vi "SR430_init.vi"(0 "GPIB address":T1, 1 "triggeLevel [V]":dbl format="%.2f", 2 "triggerSlope":bool, 3 "discriminatorLevel [V]":dbl format="%.2f", 4 "discriminatorSlope":bool, 5 "error in (no error)":errorcluster, 7 "cursorOn":bool, 9 "useExternalClock":bool) -> (14 "GPIB address out":T1, 19 "error out":errorcluster)   [LabVIEW 2015, in "SR430Driver.lvlib"]
doc: "Initializes the SR430 \n\nCopyright (C)\nGesellschaft für Schwerionenforschung, GSI\nPlanckstr. 1\n64291 Darmstadt\nGermany\n\nContact: D.Beck@gsi.de \n\nThis program is free software; you can redistribute it and/or modify it under the terms of the \nGNU General Public License as published by the Free Software Foundation; either version 2 of the license, or (at your option) any later version.\n\nThis program is distributed in the hope that it will be useful, but WITHOUT ANY WARRANTY; without even the implied warranty of MERCHANTABILITY or FITNESS FOR A PARTICULAR PURPOSE. See the GNU General License for more details (http://www.gnu.org).\n\nGesellschaft für Schwerionenforschung, GSI\nPlanckstr. 1, 64291 Darmstadt, Germany\nFor all questions and ideas contact: M.Richter@gsi.de, K.Poppensieker, H.Brand@gsi.de or D.Beck@gsi.de.\nLast update: 11-APR-2002"
uses:
  SR430Driver.lvlib
  SR430_VISA Control.ctl
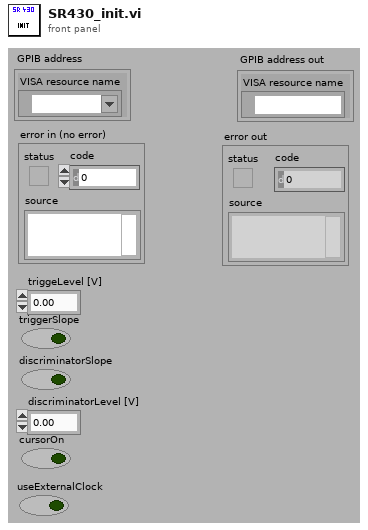
[diagram p1: front panel]
types:
  T1 = typedef "SR430Driver.lvlib/SR430_VISA Control.ctl" = cluster{"VISA resource name":refnum<visa-resource-name>}
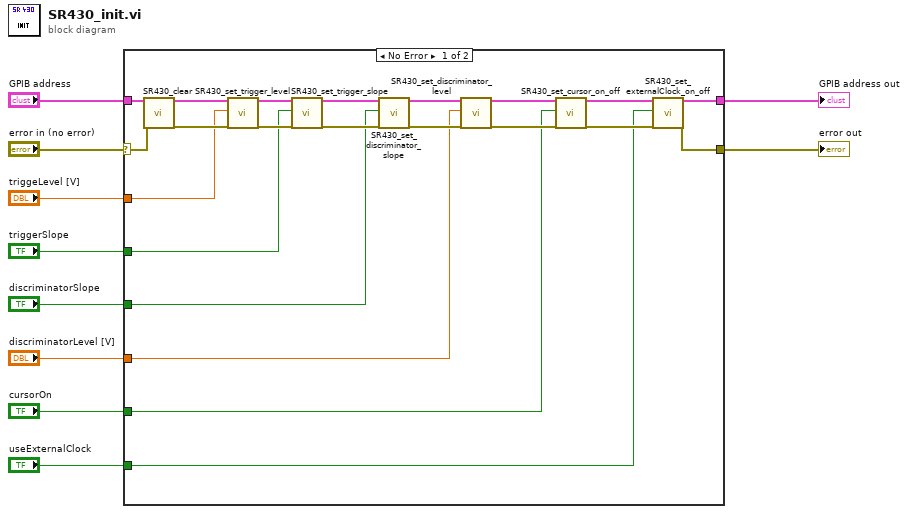
[diagram p0: block diagram]
diagram:
  n1 = case shown="No Error" "error in (no error)" {
    selector: "error in (no error)" -> [w21 w33]
    tunnel: "GPIB address" -> [w29 w34]
    tunnel: [w17 w34] -> w9
    tunnel: [w18 w33] -> w8
    tunnel: "triggeLevel [V]" -> [w16 _]
    tunnel: "triggerSlope" -> [w15 _]
    tunnel: "discriminatorSlope" -> [w14 _]
    tunnel: "discriminatorLevel [V]" -> [w13 _]
    tunnel: "cursorOn" -> [w12 _]
    tunnel: "useExternalClock" -> [w11 _]
    frame No Error {
      n2 = call "SR430_clear.vi"("address"=w29, "error in (no error)"=w21) -> ("address out"=w28:T1, "error out"=w32:errorcluster)  [unwired: 16 in]
      n3 = call "SR430_set_trigger_level.vi"("address"=w28, "triggerLevel [V]"=w16, "error in (no error)"=w32) -> ("address out"=w27:T1, "error out"=w31:errorcluster)  [unwired: 15 in]
      n4 = call "SR430_set_trigger_slope.vi"("address"=w27, "triggerSlope"=w15, "error in (no error)"=w31) -> ("address out"=w26:T1, "error out"=w30:errorcluster)  [unwired: 15 in]
      n5 = call "SR430_set_discriminator_slope.vi"("address"=w26, "discriminatorSlope"=w14, "error in (no error)"=w30) -> ("address out"=w25:T1, "error out"=w24:errorcluster)  [unwired: 15 in]
      n6 = call "SR430_set_discriminator_level.vi"("address"=w25, "discriminatorLevel [V]"=w13, "error in (no error)"=w24) -> ("address out"=w23:T1, "error out"=w22:errorcluster)  [unwired: 15 in]
      n7 = call "SR430_set_cursor_on_off.vi"("address"=w23, "cursorOn"=w12, "error in (no error)"=w22) -> ("address out"=w20:T1, "error out"=w19:errorcluster)  [unwired: 15 in]
      n8 = call "SR430_set_externalClock_on_off.vi"("address"=w20, "useExternalClock"=w11, "error in (no error)"=w19) -> ("address out"=w17:T1, "error out"=w18:errorcluster)  [unwired: 15 in]
    }
    frame Error {
    }
  }
  "error out" <- w8
  "GPIB address out" <- w9
